vi "MotorGetAxis.vi"(0 "MotorName":string, 1 "MotorData":T1[](array[typedef])) -> (2 "Axis":i32)   [LabVIEW 2009]
uses:
  Controls/MotorData.ctl
  Controls/MotorNamedPosition.ctl
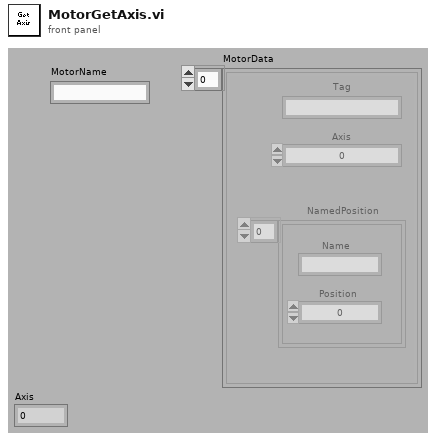
[diagram p1: front panel]
types:
  T1 = typedef "MotorData.ctl" = cluster{"Tag":string, "Axis":i32, "NamedPosition":T2[]}
  T2 = typedef "MotorNamedPosition.ctl" = cluster{"Position":i32, "Name":string}
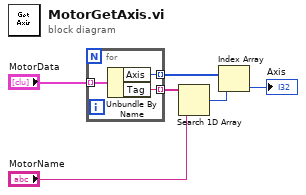
[diagram p0: block diagram]
diagram:
  n1 = for {
    tunnel: "MotorData" -> [w9] mode=indexing
    tunnel: [w8] -> w5 mode=indexing
    tunnel: [w7] -> w3 mode=indexing
    n2 = Unbundle By Name(w9) -> ("Axis"=w7:i32, "Tag"=w8:string)
  }
  n3 = Search 1D Array(1D array=w5, element="MotorName") -> (index of element=w2:i32)  [unwired: 1 out]
  n4 = Index Array(array=w3, index=w2) -> (element=→"Axis":i32)
